vi "Force Sensing V7.vi"(10 "Analog Input Pin":u8) -> (3 "Force":dbl(graph))   [LabVIEW 2013]
uses:
  <vilib>/LabVIEW Interface for Arduino/LabVIEW Interface for Arduino.lvlib
panel:
  in  "Analog Input Pin (0)":u8
  out "Force 2":dbl(graph)
  out "Voltage2":dbl(graph)
  in  "Array":dbl[](array[numeric])
  in  "Stop":bool
  out "Volatge":dbl(graph)
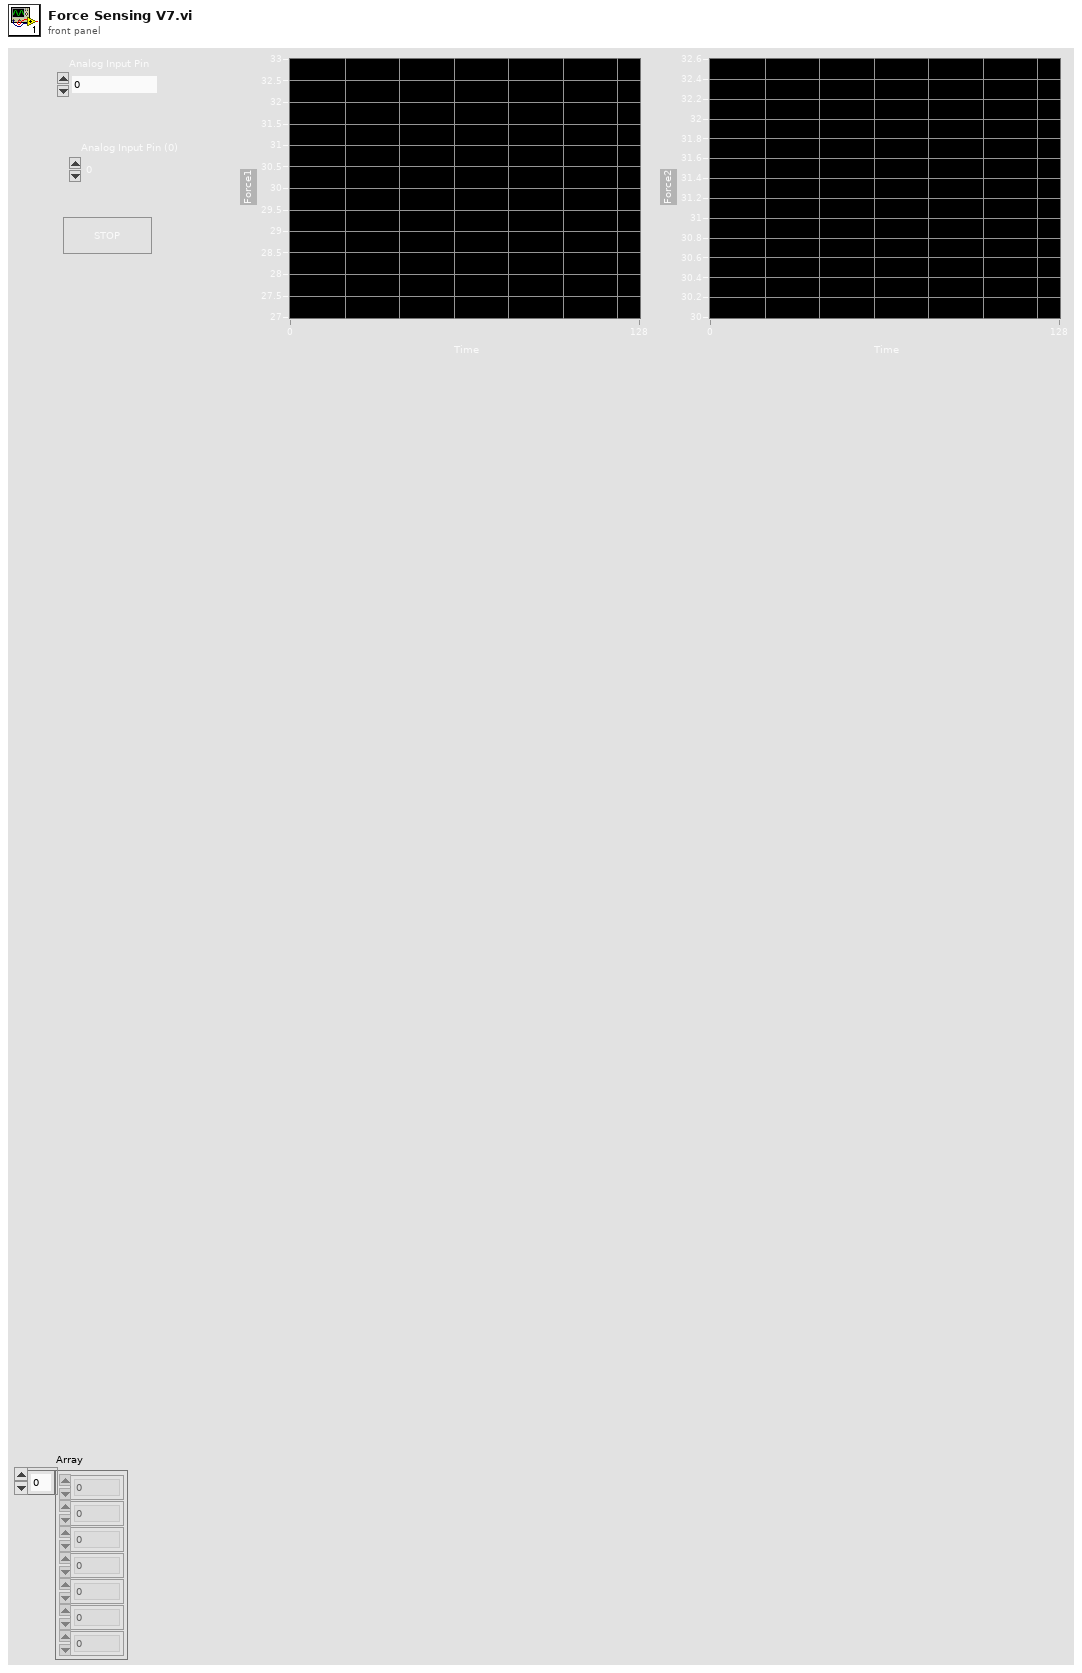
[diagram p1: front panel]
types:
  T1 = typedef "LabVIEW Interface for Arduino.lvlib/Arduino Resource.ctl" = cluster{"VISA resource":refnum<visa-resource-name>, "Board Type":T2, "Connection Type":enum8{"USB / Serial"}, "Bytes Per Packet (15)":u8}
  T2 = typedef "LabVIEW Interface for Arduino.lvlib/Board Type.ctl" = enum16{"Uno", "Dimuelanove w/Atmega 328", "Mega 2560"}
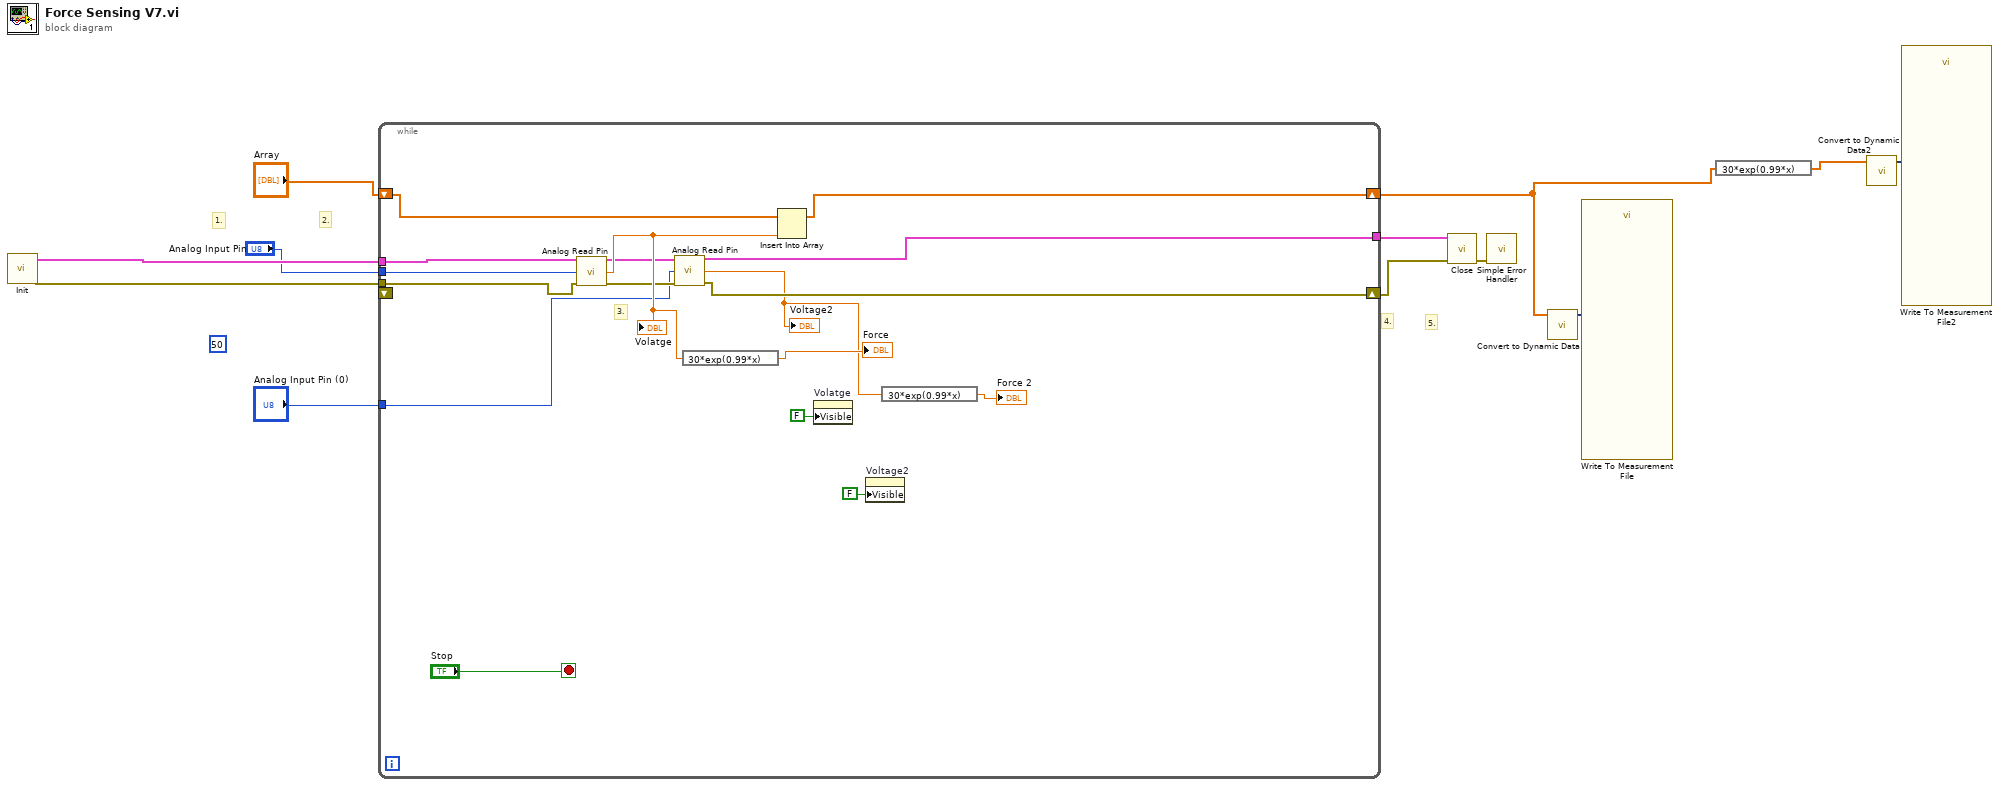
[diagram p0: block diagram]
diagram:
  (unwired) u16 50 ("Sample Rate (HZ)")
  # "5."
  # "4."
  # "2."
  # "1."
  n1 = call <vilib>:"Init.vi"() -> ("Arduino Resource"=w6:T1, "error out"=w5:errorcluster)  [unwired: 18 in]
  n2 = while {
    shift-right: [w16] -> w2
    shift-left: _ -> [_]
    shift-right: [w27] -> w9
    shift-left: "Array" -> [w28]
    tunnel: w6 -> [w22]
    tunnel: w5 -> [w21]
    tunnel: "Analog Input Pin" -> [w20]
    tunnel: [w17] -> w3
    tunnel: "Analog Input Pin (0)" -> [w13]
    stop <- "Stop" stop-if-true
    # "3."
    n3 = call <vilib>:"Analog Read Pin.vi"("Arduino Resource"=w22, "Analog Input Pin (0)"=w20, "error in"=w21) -> ("Arduino Resource"=w19:T1, "Voltage"=w23:dbl, "error out"=w18:errorcluster)  [unwired: 10 in]
    "Volatge" <- w23
    n4 = call <vilib>:"Analog Read Pin.vi"("Arduino Resource"=w19, "Analog Input Pin (0)"=w13, "error in"=w18) -> ("Arduino Resource"=w17:T1, "Voltage"=w15:dbl, "error out"=w16:errorcluster)  [unwired: 10 in]
    "Voltage2" <- w15
    n5 = expression code="30*exp(0.99*x)"(w23) -> (→"Force":dbl)
    n6 = Insert Into Array(array=w28, new element=w23) -> (w27:dbl[])  [unwired: 1 in]
    n7 = property on="Volatge" class="WFChart (strict)"("Visible"=FALSE) -> ()  [unwired: 2 in, 2 out]
    n8 = property on="Voltage2" class="WFChart (strict)"("Visible"=FALSE) -> ()  [unwired: 2 in, 2 out]
    n9 = expression code="30*exp(0.99*x)"(w15) -> (→"Force 2":dbl)
  }
  n10 = call <vilib>:"Close.vi"("Arduino Resource"=w3, "error in"=w2) -> ("error out"=w12:errorcluster)  [unwired: 13 in]
  n11 = call <vilib>:"Simple Error Handler.vi"("error in (no error)"=w12) -> ()  [unwired: 4 in, 5 out]
  n12 = call "Convert to Dynamic Data"("Array"=w9) -> ("Dynamic Data Type"=w10:dynamicdata)  [unwired: 3 in]
  n13 = call "Write To Measurement File"("Signals"=w10) -> ()  [unwired: 16 in, 3 out]
  n14 = expression code="30*exp(0.99*x)"(w9) -> (w8:dbl[])
  n15 = call "Convert to Dynamic Data2"("Array"=w8) -> ("Dynamic Data Type"=w7:dynamicdata)  [unwired: 3 in]
  n16 = call "Write To Measurement File2"("Signals"=w7) -> ()  [unwired: 16 in, 3 out]
